vi "一组模拟量CAN切换开关.vi"(9 "第几组数据":u8) -> (2 "成功？":bool)   [LabVIEW 2010]
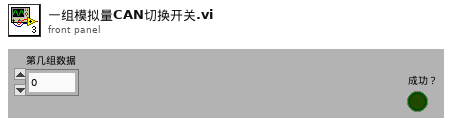
[diagram p1: front panel]
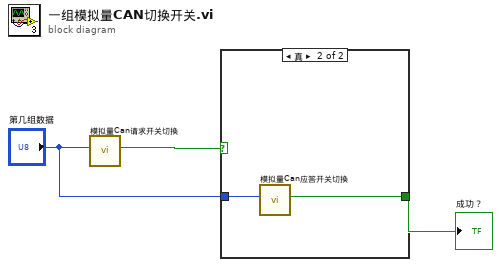
[diagram p0: block diagram]
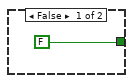
[diagram p2: hidden frame]
diagram:
  n1 = call "模拟量Can请求开关切换.vi"("第几组"="第几组数据") -> ("发送成功?"=w2:bool)  [unwired: 10 in]
  n2 = case shown="真" w2 {
    tunnel: "第几组数据" -> [_ w6]
    tunnel: [FALSE w5] -> w1
    frame False {
    }
    frame True {
      n3 = call "模拟量Can应答开关切换.vi"("第几组"=w6) -> ("成功？"=w5:bool)  [unwired: 9 in, 1 out]
    }
  }
  "成功？" <- w1
